vi "DB_Read_Write.vi"(7 "Write Data":variant[][](array[variant]), 8 "error in (no error)":errorcluster, 9 "DB Name":string="MMUM_ST05", 10 "Enum":enum16{"Read", "Write"}(ring), 11 "Table Nmae":string="IO_LIST") -> (0 "error out":errorcluster, 2 "Header columns":string[](array[string]), 3 "Read data":variant[][](array[variant]))   [LabVIEW 2015]
uses:
  <vilib>/addons/database/Connection.llb/DB Tools Open Connec (String).vi
  <vilib>/addons/database/NI_Database_API.lvlib
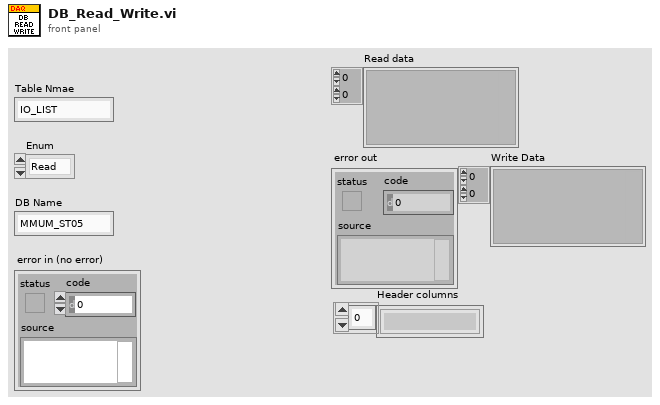
[diagram p1: front panel]
types:
  T1 = typedef "NI_Database_API.lvlib/Conn ObjectReference.ctl" = refnum<k1>
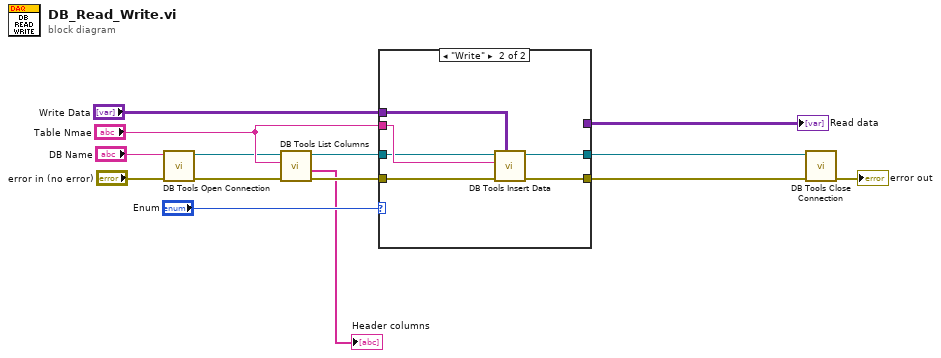
[diagram p0: block diagram]
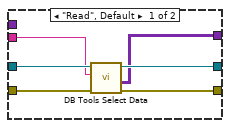
[diagram p2: hidden frame]
diagram:
  n1 = call-poly <vilib>:"DB Tools Open Connection.vi"("error in (no error)"="error in (no error)", "connection information"="DB Name") -> ("error out"=w3:errorcluster, "connection reference"=w5:T1)  [unwired: 6 in]
  n2 = call <vilib>:"DB Tools List Columns.vi"("error in (no error)"=w3, "table"="Table Nmae", "connection reference"=w5) -> ("error out"=w2:errorcluster, "columns"=→"Header columns":string[], "connection reference out"=w4:T1)  [unwired: 1 in, 1 out]
  n3 = case shown="\"Write\"" "Enum" {
    tunnel: w4 -> [w20 w22]
    tunnel: w2 -> [w19 w21]
    tunnel: [w18 w26] -> w10
    tunnel: [w17 w25] -> w9
    tunnel: "Table Nmae" -> [w16 w23]
    tunnel: [w15 _] -> w11
    tunnel: "Write Data" -> [_ w24]
    frame "Read", Default {
      n4 = call <vilib>:"DB Tools Select Data.vi"("error in (no error)"=w19, "table"=w16, "connection reference"=w20) -> ("error out"=w17:errorcluster, "data"=w15:variant[][], "connection reference out"=w18:T1)  [unwired: 3 in]
    }
    frame "Write" {
      n5 = call <vilib>:"DB Tools Insert Data.vi"("data"=w24, "error in (no error)"=w21, "table"=w23, "connection reference"=w22) -> ("error out"=w25:errorcluster, "connection reference out"=w26:T1)  [unwired: 6 in]
    }
  }
  "Read data" <- w11
  n6 = call <vilib>:"DB Tools Close Connection.vi"("error in (no error)"=w9, "connection reference"=w10) -> ("error out"=→"error out":errorcluster)  [unwired: 5 in]
